vi "SC TCP Open Sequence Command.vi"(8 "error in (no error)":errorcluster, 9 "timeout (ms)":i32=10000, 10 "Sequence to run (full path)":path, 11 "TCP Network Connection in":refnum<k5>) -> (0 "error out":errorcluster, 3 "Sequence Opened":bool)   [LabVIEW 2018]
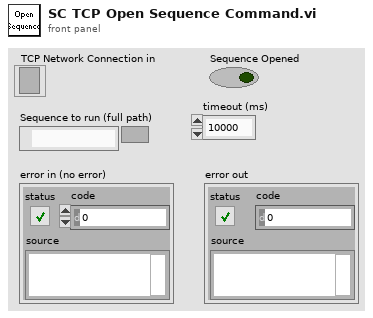
[diagram p1: front panel]
types:
  T1 = cluster{"cmdCompleted":bool, "returnType":string, "errorType":string, "errorDescription":string, "originalCommand":string, "resolvedCommand":string}
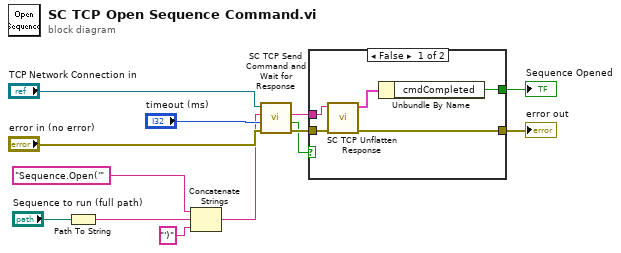
[diagram p0: block diagram]
diagram:
  n1 = Path To String(path="Sequence to run (full path)") -> (string=w5:string)
  n2 = Concatenate Strings("Sequence.Open('", w5, "')") -> (w7:string)
  n3 = call "SC TCP Send Command and Wait for Response.vi"("error in (no error)"="error in (no error)", "timeout (10000 ms)"="timeout (ms)", "Command"=w7, "TCP Network Connection in"="TCP Network Connection in") -> ("error out"=w10:errorcluster, "Timed Out"=w2:bool, "Response"=w1:string)  [unwired: 4 in, 1 out]
  n4 = case shown="False" w2 {
    tunnel: [w18 w19] -> w12
    tunnel: [w17 _] -> w11
    tunnel: w1 -> [w15 _]
    tunnel: w10 -> [w14 w19]
    frame False {
      n5 = call "SC TCP Unflatten Response.vi"("error in"=w14, "Response JSON"=w15) -> ("error out"=w18:errorcluster, "Response Details"=w16:T1)  [unwired: 8 in]
      n6 = Unbundle By Name(w16) -> ("cmdCompleted"=w17:bool)
    }
    frame True {
      # "Timed out"
    }
  }
  "error out" <- w12
  "Sequence Opened" <- w11
